vi "rotary_encoder_lookup.vi"(11 "Code from Encoder":u8) -> (0 "angle (deg)":dbl)   [LabVIEW 2019]
panel:
  out "Code from Encoder 2":u8
  out "Code from Encoder":u8(graph)
  out "Position code":i32(graph)
  out "Waveform Graph":u8[](graph)
  out "angle (deg)":dbl(graph)
  out "Position code":i32
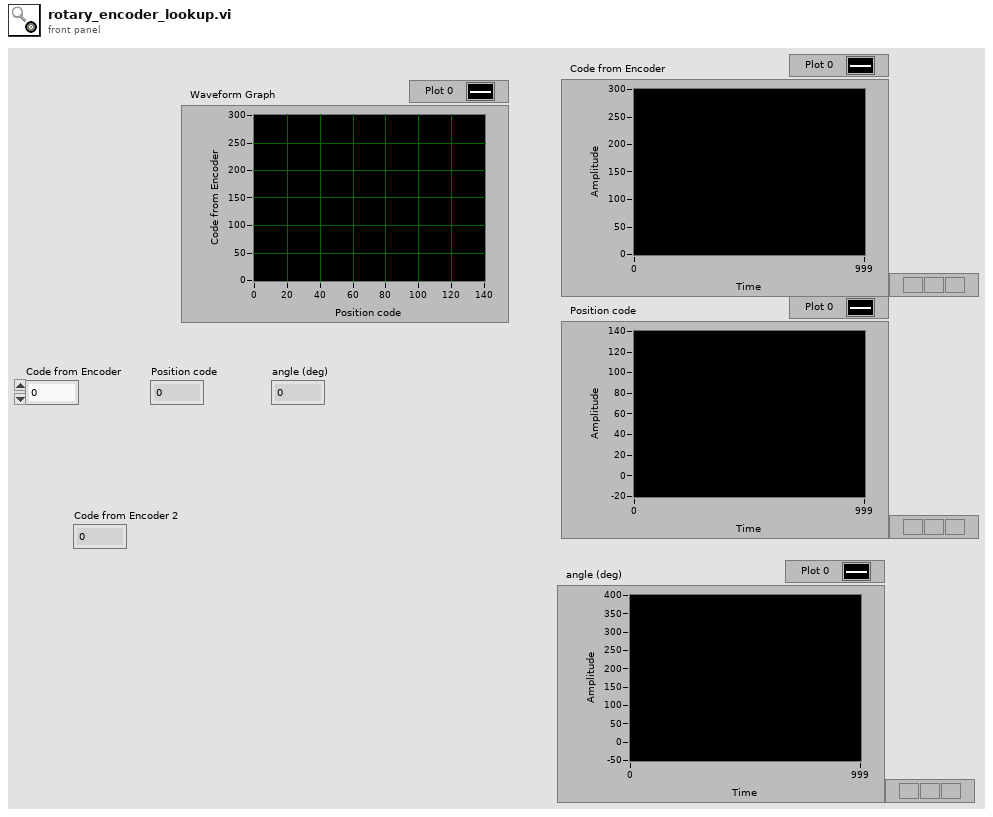
[diagram p1: front panel]
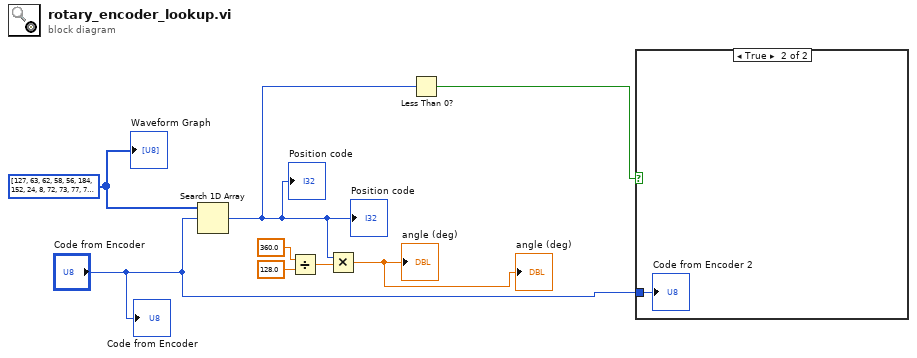
[diagram p0: block diagram]
diagram:
  w4 = u8[] [127, 63, 62, 58, 56, 184, 152, 24, 8, 72, 73, 77, 79, 15, 47, 175, 191, 159, 31, 29, 28, 92, 76, 12, 4, 36, 164, 166, 167, 135, 151, 215, 223, 207, 143, 142, 14, 46, 38, 6, 2, 18, 82, 83, 211, 195, 203, 235, 239, 231, 199, 71, 7, 23, 19, 3, 1, 9, 41, 169, 233, 225, 229, 245, 247, 243, 227, 163, 131, 139, 137, 129, 128, 132, 148, 212, 244, 240, 242, 250, 251, 249, 241, 209, 193, 197, 196, 192, 64, 66, 74, 106, 122, 120, 121, 125, 253, 252, 248, 232, 224, 226, 98, 96, 32, 33, 37, 53, 61, 60, 188, 190, 254, 126, 124, 116, 112, 113, 49, 48, 16, 144, 146, 154, 158, 30, 94, 95] ("transposed array")
  n1 = Search 1D Array(1D array=w4, element="Code from Encoder") -> (index of element=w3:i32)  [unwired: 1 in]
  "Position code" <- w3
  "Position code" <- w3
  n2 = Divide(x=360.0 ("y"), y=128.0) -> (x/y=w6:dbl)
  n3 = Multiply(x=w3, y=w6) -> (x*y=→"angle (deg)" →"angle (deg)":dbl)
  n4 = Less Than 0?(x=w3) -> (x < 0?=w2:bool)
  n5 = case shown="True" w2 {
    tunnel: "Code from Encoder" -> [_ w9]
    frame False {
    }
    frame True {
      "Code from Encoder 2" <- w9
    }
  }
  "Waveform Graph" <- w4
  "Code from Encoder" <- "Code from Encoder"
